vi "Map.vi"(6 "B max":dbl, 8 "B min":dbl, 9 "A max":dbl, 10 "A min":dbl, 11 "A":dbl) -> (3 "B":dbl)   [LabVIEW 2018]
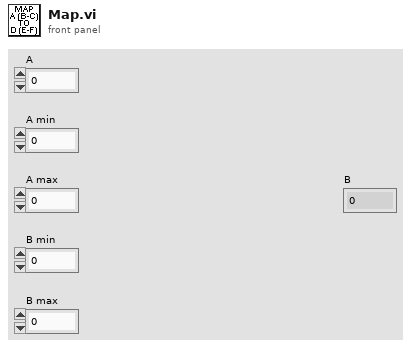
[diagram p1: front panel]
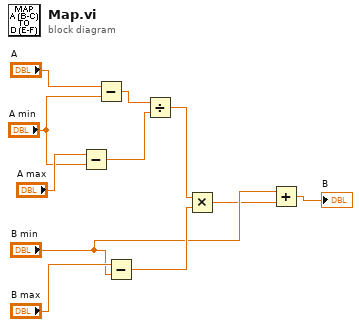
[diagram p0: block diagram]
diagram:
  n1 = Subtract(x="A max", y="A min") -> (x-y=w7:dbl)
  n2 = Subtract(x="A", y="A min") -> (x-y=w10:dbl)
  n3 = Subtract(x="B max", y="B min") -> (x-y=w4:dbl)
  n4 = Divide(x=w10, y=w7) -> (x/y=w5:dbl)
  n5 = Multiply(x=w5, y=w4) -> (x*y=w2:dbl)
  n6 = Add(x="B min", y=w2) -> (x+y=→"B":dbl)
